vi "Parse Full ISO 8601 UTC.vi"(8 "error in (no error)":errorcluster, 11 "full ISO 8601 UTC":string) -> (0 "error out":errorcluster, 3 "Time Stamp":timestamp)   [LabVIEW 2018, in "XML Config.lvlib"]
uses:
  XML Config/XML Config.lvlib
  <vilib>/Utility/miscctls.llb/LVDateTimeRec.ctl
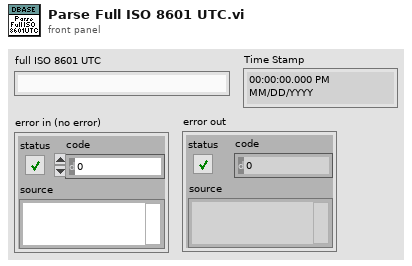
[diagram p1: front panel]
types:
  T1 = typedef "LVDateTimeRec.ctl" = cluster{"fractional second":dbl, "second":i32, "minute":i32, "hour":i32, "day of month":i32, "month":i32, "year":i32, "day of week":i32, "day of year":i32, "DST":i32}
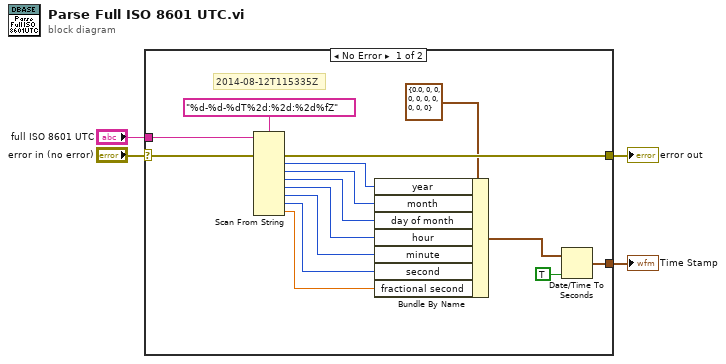
[diagram p0: block diagram]
diagram:
  n1 = case shown="No Error" "error in (no error)" {
    selector: "error in (no error)" -> [w18 w20]
    tunnel: [w17 w20] -> w3
    tunnel: "full ISO 8601 UTC" -> [w19 _]
    tunnel: [w12 _] -> w1
    frame No Error {
      # "2014-08-12T115335Z"
      n2 = Scan From String(format string="%d-%d-%dT%2d:%2d:%2d%fZ", input string=w19, error in=w18) -> (error out=w17:errorcluster, output 1=w11:i32, output 2=w10:i32, output 3=w9:i32, output 4=w8:i32, output 5=w7:i32, output 6=w6:i32, output 7=w5:dbl)  [unwired: 8 in, 2 out]
      n3 = Bundle By Name(cluster=T1 {"fractional second"=0.0, "second"=0, "minute"=0, "hour"=0, "day of month"=0, "month"=0, "year"=0, "day of week"=0, "day of year"=0, "DST"=0} ("date time rec"), "year"=w11, "month"=w10, "day of month"=w9, "hour"=w8, "minute"=w7, "second"=w6, "fractional second"=w5) -> (w13:T1)
      n4 = Date/Time To Seconds(1:TRUE ("is UTC (F)"), 2:w13) -> (0:w12:timestamp)
    }
    frame Error {
    }
  }
  "Time Stamp" <- w1
  "error out" <- w3
